vi "Create.vi"(8 "error in (no error)":errorcluster, 11 "Model":T1) -> (0 "error out":errorcluster, 3 "Text Recognizer":refnum<class "Text Recognizer.lvclass">)   [LabVIEW 2020, in "feature_detection.lvlib" / "Text Recognizer.lvclass"]
uses:
  Text Recognizer.lvclass
  Model.ctl
  Mode.ctl
  common/Image Size (Integer).ctl
  common/Object Point (Float).ctl
  Text Recognizer.lvclass/Text Recognizer.ctl
  common/common.lvlib
  common/bin/gartoolkit_32-1.dll
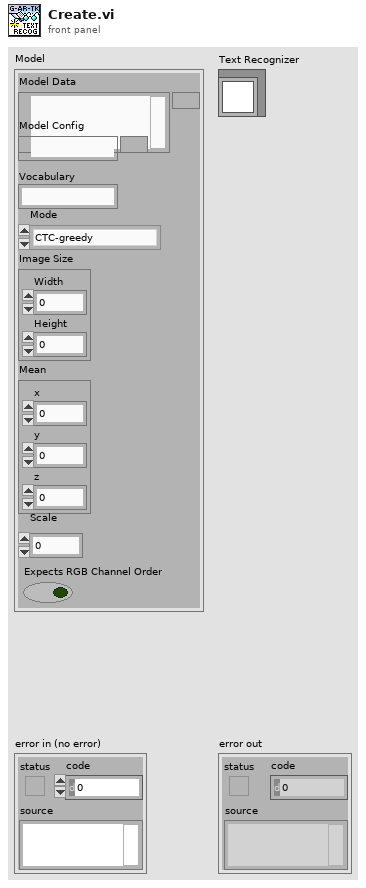
[diagram p1: front panel]
types:
  T1 = typedef "feature_detection.lvlib/Text Recognizer.lvclass/Model.ctl" = cluster{"Model Data":path, "Model Config":path, "Vocabulary":string, "Mode":T2, "Image Size":T3, "Mean":T4, "Scale":dbl, "Expects RGB Channel Order":bool}
  T2 = typedef "feature_detection.lvlib/Text Recognizer.lvclass/Mode.ctl" = enum8{"CTC-greedy", "CTC-prefix-beam-search"}
  T3 = typedef "common.lvlib/Image Size (Integer).ctl" = cluster{"Width":u16, "Height":u16}
  T4 = typedef "common.lvlib/Object Point (Float).ctl" = cluster{"x":dbl, "y":dbl, "z":dbl}
  T5 = cluster{"String":string, "String":string, "Vocabulary":string, "Mode":T2, "Image Size":T3, "Mean":T4, "Scale":dbl, "Expects RGB Channel Order":bool}
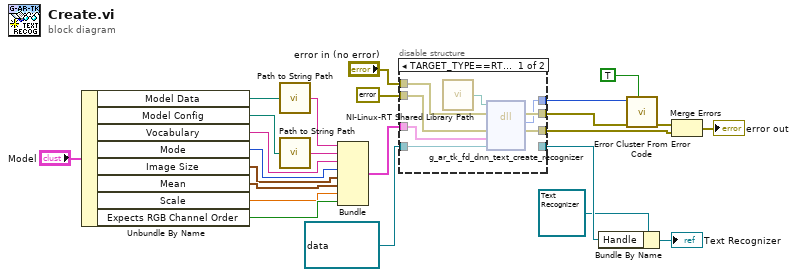
[diagram p0: block diagram]
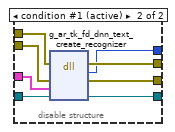
[diagram p2: hidden frame]
diagram:
  n1 = Unbundle By Name("Model") -> ("Model Data"=w5:path, "Model Config"=w2:path, "Vocabulary"=w6:string, "Mode"=w7:T2, "Image Size"=w8:T3, "Mean"=w9:T4, "Scale"=w10:dbl, "Expects RGB Channel Order"=w11:bool)
  n2 = call "Path to String Path.vi"("Path"=w5) -> ("String"=w4:string)
  n3 = call "Path to String Path.vi"("Path"=w2) -> ("String"=w3:string)
  n4 = Bundle("String"=w4, "String"=w3, "Vocabulary"=w6, "Mode"=w7, "Image Size"=w8, "Mean"=w9, "Scale"=w10, "Expects RGB Channel Order"=w11) -> (w1:T5)  [unwired: 1 in]
  n5 = disable-structure "Conditional Disable Structure" shown="TARGET_TYPE==RT&&OS==Linux" {
    disable-tunnel: "error in (no error)" -> [w26 w40]
    disable-tunnel: errorcluster {"status"=FALSE, "code"=0, "source"=""} ("error constant") -> [w25 w39]
    disable-tunnel: refnum<data-value> refnum ("EDVR") -> [w27 w38]
    disable-tunnel: [w32 w37] -> w21
    disable-tunnel: [w30 w36] -> w20
    disable-tunnel: [_ w35] -> w19
    disable-tunnel: [w31 w34] -> w18
    disable-tunnel: w1 -> [w28 w33]
    frame condition #0 {
      n6 = call "NI-Linux-RT Shared Library Path.vi"() -> ("Path"=w29:path)
      n7 = dll-call lib="?" fn="g_ar_tk_fd_dnn_text_create_recognizer" ("g_ar_toolkit.*.*:g_ar_tk_capture_context_create")(path in=w29, error in=w26, w25, "model"=w28, "EDVR"=w27) -> (error out=w32:errorcluster, "return type"=w30:i32, w31:errorcluster)  [unwired: 3 in, 1 out]
    }
    frame condition #1 (active) {
      n8 = dll-call lib="C:/serenial/lib/g-augmented-reality-toolkit/LabVIEW/common/bin/gartoolkit_*-1.*" fn="g_ar_tk_fd_dnn_text_create_recognizer" ("g_ar_toolkit.*.*:g_ar_tk_capture_context_create")(error in=w40, "error_cluster"=w39, "model"=w33, "EDVR"=w38) -> (error out=w37:errorcluster, "return type"=w36:i32, "error_cluster"=w34:errorcluster, "EDVR"=w35:refnum<data-value>)  [unwired: 3 in, 1 out]
    }
  }
  n9 = Bundle By Name(cluster=refnum<class "Text Recognizer.lvclass"> refnum ("Text Detector in"), "Handle"=w19) -> (→"Text Recognizer":refnum<class "Text Recognizer.lvclass">)
  n10 = call <vilib>:"Error Cluster From Error Code.vi"("show call chain? (False)"=TRUE, "error in (no error)"=w21, "error code (0)"=w20) -> ("error out"=w24:errorcluster)  [unwired: 6 in]
  n11 = Merge Errors(w24, w18) -> (→"error out":errorcluster)
